vi "Converter_average_fom_sum_array.vi"(11 "Sum array in":T1) -> (3 "Average array out":dbl[][](array[numeric]))   [LabVIEW 2013]
uses:
  Sum_array_for_avg_baseline.ctl
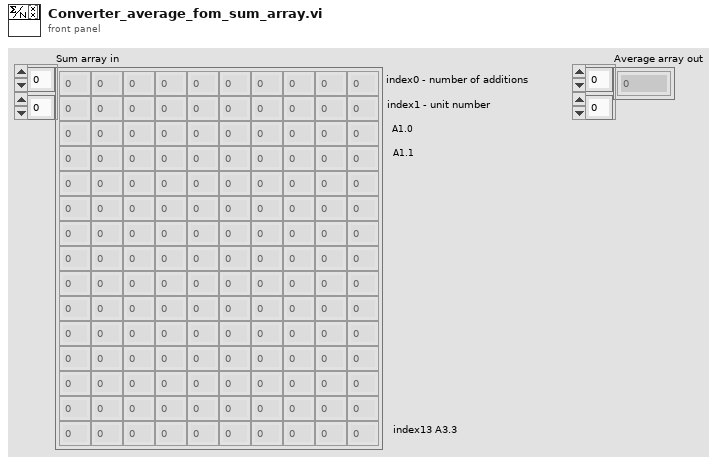
[diagram p1: front panel]
types:
  T1 = typedef "Sum_array_for_avg_baseline.ctl" = dbl[][]
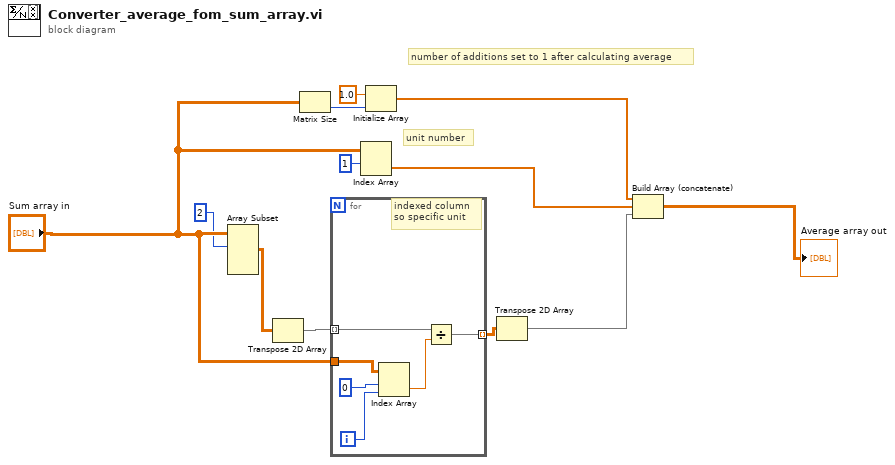
[diagram p0: block diagram]
diagram:
  # "number of additions set to 1 after calculating average"
  # "unit number"
  n1 = Array Subset(array="Sum array in", index (row)=2 ("index")) -> (w2:T1)  [unwired: 3 in]
  n2 = Transpose 2D Array(2D array=w2) -> (transposed array=w3:T1)
  n3 = Matrix Size(0:"Sum array in") -> (2:w5:i32)  [unwired: 1 out]
  n4 = for {
    tunnel: w3 -> [w18] mode=indexing
    tunnel: [w17] -> w4 mode=indexing
    tunnel: "Sum array in" -> [w15]
    i -> [w13]
    # "indexed column\nso specific unit"
    n5 = Index Array(array=w15, index (row)=0, index (col)=w13) -> (element=w16:dbl)
    n6 = Divide(x=w18, y=w16) -> (x/y=w17:dbl[])
  }
  n7 = Index Array(array="Sum array in", index (row)=1) -> (element=w10:dbl[])  [unwired: 1 in]
  n8 = Initialize Array(1.0 ("element"), w5) -> (w11:dbl[])
  n9 = Transpose 2D Array(2D array=w4) -> (transposed array=w9:dbl[][])
  n10 = Build Array (concatenate)(w11, w10, w9) -> (→"Average array out":dbl[][])
